vi "Get Column Name.vi"(8 "error in (no error)":errorcluster, 11 "Basic Column Configuration in":refnum<class "Base Column Configuration.lvclass">) -> (0 "error out":errorcluster, 2 "Column Name":string, 3 "Basic Column Configuration out":refnum<class "Base Column Configuration.lvclass">)   [LabVIEW 2020, in "Column Interfaces.lvlib" / "Base Column Configuration.lvclass"]
uses:
  Base Column Configuration.lvclass
  Base Column Configuration.lvclass/Base Column Configuration.ctl
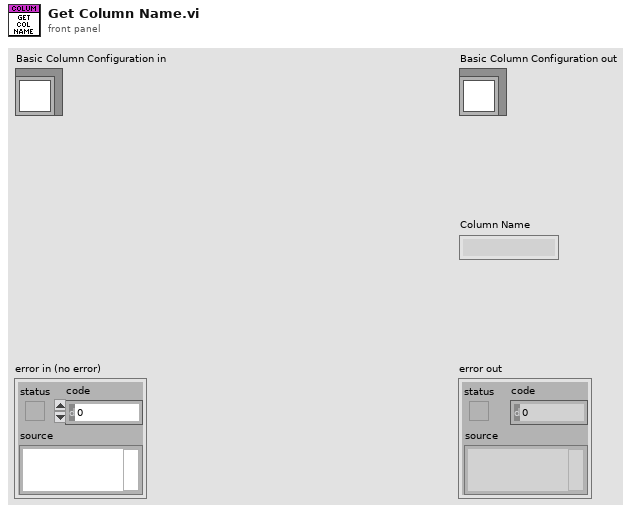
[diagram p1: front panel]
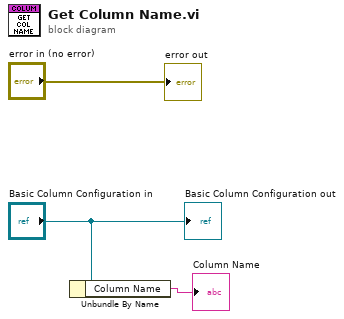
[diagram p0: block diagram]
diagram:
  n1 = Unbundle By Name("Basic Column Configuration in") -> ("Column Name"=→"Column Name":string)
  "error out" <- "error in (no error)"
  "Basic Column Configuration out" <- "Basic Column Configuration in"
